vi "ReadMaxAmp.vi"(8 "error in (no error)":errorcluster, 9 "Channel":dbl, 11 "Simulated Scope in":refnum<class "Simulated Scope.lvclass">) -> (0 "error out":errorcluster, 1 "Amplitude":dbl, 3 "Simulated Scope out":refnum<class "Simulated Scope.lvclass">)   [LabVIEW 2026, in "Simulated Scope.lvclass"]
uses:
  Simulated Scope.lvclass
panel:
  out "Count":dbl
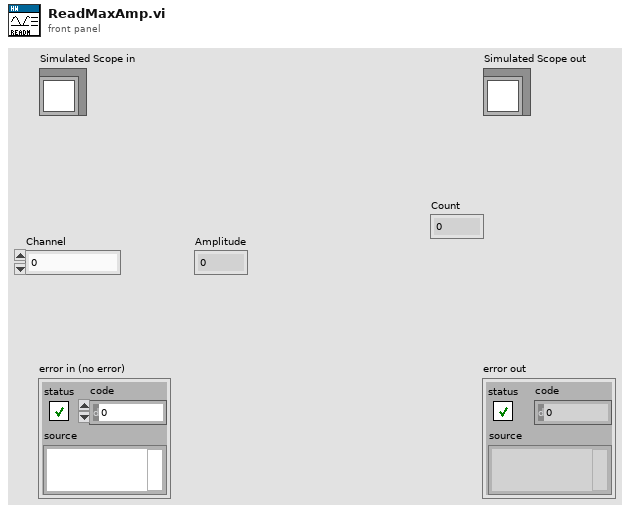
[diagram p1: front panel]
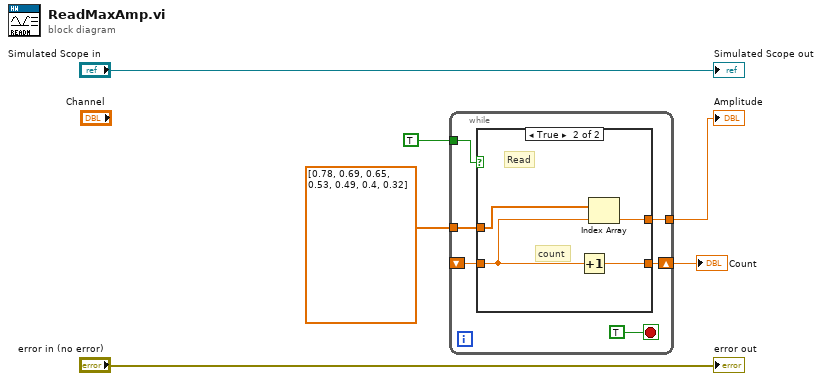
[diagram p0: block diagram]
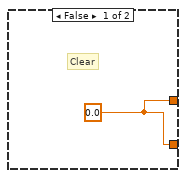
[diagram p2: hidden frame]
diagram:
  n1 = while {
    shift-right: [w11] -> w4
    shift-left: _ -> [w10]
    tunnel: dbl[] [0.78, 0.69, 0.65, 0.53, 0.49, 0.4, 0.32] ("Freq Amp Array") -> [w9]
    tunnel: [w8] -> w2
    tunnel: TRUE -> [w7]
    stop <- TRUE stop-if-true
    n2 = case shown="True" w7 {
      tunnel: [w13 w17] -> w11
      tunnel: w10 -> [_ w15]
      tunnel: w9 -> [_ w16]
      tunnel: [w13 w14] -> w8
      frame False {
        w13 = 0.0 ("Amplitude")
        # "Clear"
      }
      frame True {
        # "count"
        # "Read"
        n3 = Increment(x=w15) -> (x+1=w17:dbl)
        n4 = Index Array(array=w16, index=w15) -> (element=w14:dbl)
      }
    }
  }
  "Amplitude" <- w2
  "Count" <- w4
  "error out" <- "error in (no error)"
  "Simulated Scope out" <- "Simulated Scope in"
